vi "Translate.vi"(10 "Message In":refnum<class "MSG.lvclass">, 11 "Translator in":refnum<class "LabelPrefix.lvclass">) -> (2 "Translated Message":refnum<class "MSG.lvclass">, 3 "Translator out":refnum<class "LabelPrefix.lvclass">)   [LabVIEW 2011, in "Messenging.lvlib" / "LabelPrefix.lvclass"]
uses:
  LabelPrefix.lvclass
  TextVarientMessage/MSG.lvclass
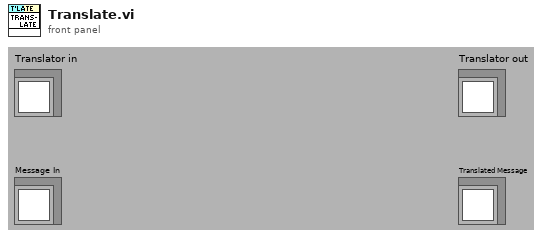
[diagram p1: front panel]
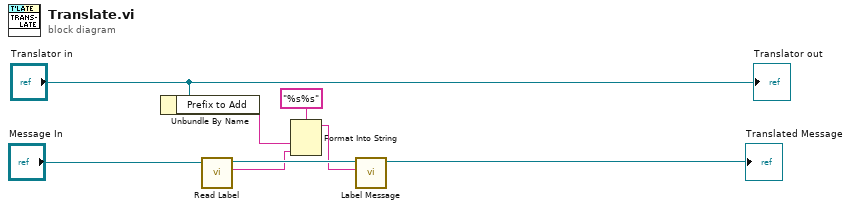
[diagram p0: block diagram]
diagram:
  n1 = Unbundle By Name("Translator in") -> ("Prefix to Add"=w4:string)
  n2 = call-dynamic "Read Label.vi"("Message"="Message In") -> ("Label"=w3:string, "Message"=w5:refnum<class "MSG.lvclass">)  [unwired: 1 in, 8 out]
  n3 = Format Into String(format string="%s%s", w4, w3) -> (resulting string=w1:string)  [unwired: 2 in, 1 out]
  n4 = call-dynamic "Label Message.vi"("Label"=w1, "Message"=w5) -> ("Message"=→"Translated Message":refnum<class "MSG.lvclass">)  [unwired: 1 in, 8 out]
  "Translator out" <- "Translator in"
